vi "GDSArray_RemoveEmptyStringElements.vi"(2 "String array":string[](array[string])) -> (16 "String array out":string[](array[string]))   [LabVIEW 2012]
doc: "Removes empty strings from the array."
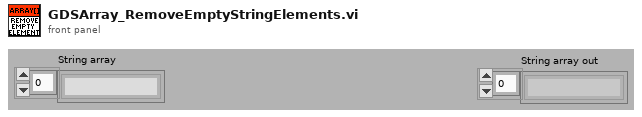
[diagram p1: front panel]
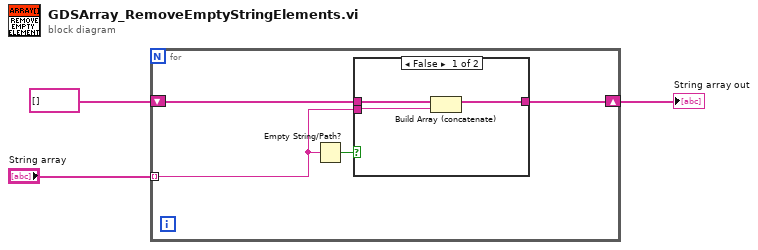
[diagram p0: block diagram]
diagram:
  n1 = for {
    tunnel: "String array" -> [w5] mode=indexing
    shift-right: [w4] -> w1
    shift-left: string[] [] ("Array Constant") -> [w7]
    n2 = Empty String/Path?(string/path=w5) -> (empty?=w6:bool)
    n3 = case shown="False" w6 {
      tunnel: w7 -> [w10 w11]
      tunnel: w5 -> [w9 _]
      tunnel: [w8 w11] -> w4
      frame False {
        n4 = Build Array (concatenate)(w10, w9) -> (w8:string[])
      }
      frame True {
      }
    }
  }
  "String array out" <- w1
